vi "CheckDFBlockTime.vi"(7 "qbus in":refnum<class "Qbus.lvclass">, 8 "error in (no error)":errorcluster, 10 "DataGroup":string, 11 "Map":T1) -> (0 "error out":errorcluster)   [LabVIEW 2017, in "DataFlow.lvlib"]
uses:
  <vilib>/addons/InsightCM/Devices/Shared/Common/DataFlow/DataFlow.lvlib
  <vilib>/addons/PointValueMap/controls/PointMap.ctl
  <vilib>/addons/Qbus/Qbus.lvclass
  <vilib>/addons/PointValueMap/subVIs/Point_Read_double.vi
  <vilib>/addons/PointValueMap/subVIs/Point_Read_i32.vi
  <vilib>/addons/TraceLogger/TraceLogger.lvlib
  <vilib>/addons/PointValueMap/PointValueMap.lvlib
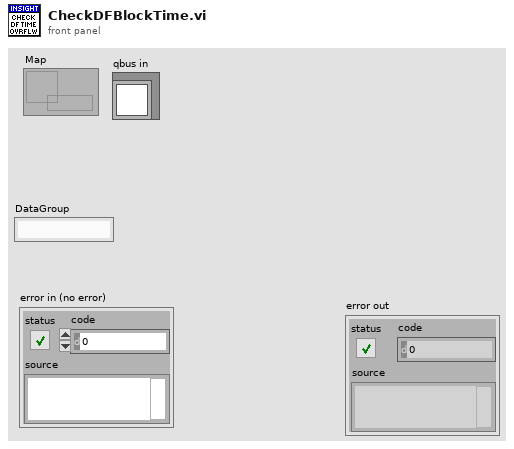
[diagram p1: front panel]
types:
  T1 = typedef "PointValueMap.lvlib/PointMap.ctl" = refnum<data-value>
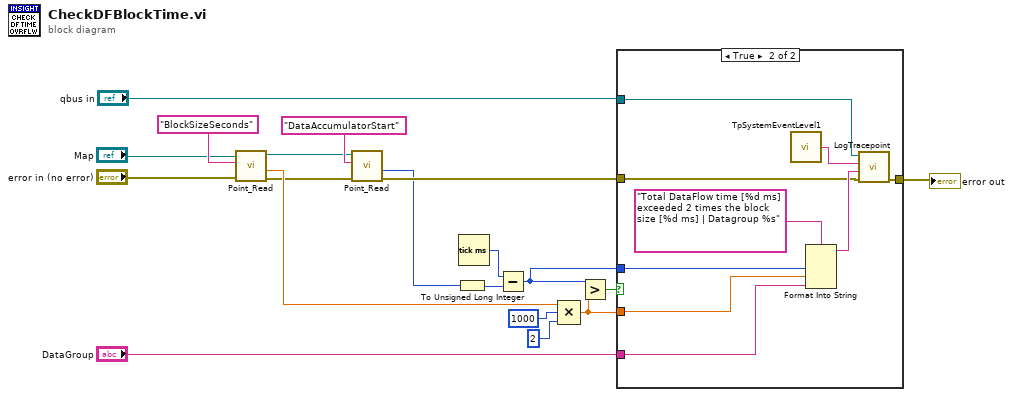
[diagram p0: block diagram]
diagram:
  n1 = call-poly <vilib>:"Point_Read.vi"("Error In"="error in (no error)", "Tag"="BlockSizeSeconds", "Map"="Map") -> ("Error Out"=w6:errorcluster, "Value"=w10:dbl, "Map Out"=w5:T1)  [unwired: 3 in, 3 out]
  n2 = call-poly <vilib>:"Point_Read.vi"("Error In"=w6, "Tag"="DataAccumulatorStart", "Map"=w5) -> ("Error Out"=w4:errorcluster, "Value"=w3:i32)  [unwired: 3 in, 4 out]
  n3 = To Unsigned Long Integer(number=w3) -> (unsigned 32bit integer=w7:u32)
  n4 = Tick Count (ms)() -> (millisecond timer value=w9:u32)
  n5 = Subtract(x=w9, y=w7) -> (x-y=w2:u32)
  n6 = Compound Arithmetic op=MULTIPLY(w10, u32 1000 ("x-y"), u32 2 ("x-y")) -> (w17:dbl)
  n7 = Greater?(x=w2, y=w17) -> (0:w18:bool)
  n8 = case shown="True" w18 {
    tunnel: [w20 w29] -> w16
    tunnel: w2 -> [_ w26]
    tunnel: w17 -> [_ w25]
    tunnel: "qbus in" -> [_ w23]
    tunnel: "DataGroup" -> [_ w22]
    tunnel: w4 -> [w20 w21]
    frame False {
    }
    frame True {
      n9 = call <vilib>:"TpSystemEventLevel1.vi"() -> ("tracepoint name"=w28:string)  [unwired: 5 in]
      n10 = Format Into String(format string="Total DataFlow time [%d ms] exceeded 2 times the block size [%d ms] | Datagroup %s", w26, w25, w22) -> (resulting string=w24:string)  [unwired: 2 in, 1 out]
      n11 = call <vilib>:"LogTracepoint.vi"("error in (no error)"=w21, "log string"=w24, "tracepoint"=w28, "qbus in"=w23) -> ("error out"=w29:errorcluster)  [unwired: 6 in, 1 out]
    }
  }
  "error out" <- w16
